vi "RFSA List Mode Frequency Sweep.vi"() -> ()   [LabVIEW 2017]
doc: "Demonstrates the basics of RF list mode using the RF vector signal analyzer. The example shows how to configure the device for RF list mode and how to create a configuration list and configuration list steps. It uses RF list mode to vary the I/Q carrier frequency and reference level across different steps that advance on a hardware timer edge."
uses:
  <instrlib>/niRFSA/niRFSA.llb/niRFSA Acquisition Types.ctl
  <instrlib>/niRFSA/niRFSA.llb/niRFSA Trigger Terminals.ctl
  <vilib>/Utility/error.llb/DialogType.ctl
  <vilib>/Analysis/1siggen.llb/Ramp Pattern by Samples.vi
  <instrlib>/niRFSA/niRFSA.llb/niRFSA Configure Digital Edge Advance Trigger.vi
  <instrlib>/niRFSA/niRFSA.llb/niRFSA Fetch IQ (1D Complex Cluster NRec 1Chan).vi
  <instrlib>/niRFSA/niRFSA.llb/niRFSA Get IQ Components (Complex Cluster).vi
  <vilib>/Analysis/NI_AALBase.lvlib
panel:
  in  "Frequency Settling (s)":dbl=0.006 format="%#_6p"
  in  "Reference Level (dBm)":dbl caption="Reference Level Ramp Start (dBm)" format="%.2g"
  out "Q Data":cluster{"t0":dbl, "dt":dbl, "Y":dbl[]}[](graph)
  out "I Data":cluster{"t0":dbl, "dt":dbl, "Y":dbl[]}[](graph)
  in  "Timer Event Interval (s)":dbl=0.001 format="%#_6p"
  in  "Carrier Frequency Ramp Start (Hz)":dbl=990000000.0 format="%#.3p"
  in  "Carrier Frequency Ramp End (Hz)":dbl=1010000000.0 format="%#.3p"
  in  "Number of Steps/Records":dbl=10.0
  in  "Samples per Step/Record":dbl=10000.0 format="%#_6p"
  in  "IQ Rate (S/s)":dbl=10000000.0 format="%#_6p"
  in  "Resource Name":refnum<k15>="RFSA"
  # "Overview: Demonstrates the basics of RF list mode using the RF vector signal analyzer. \nRequirements: NI-RFSA\nInstructions:\n1. Change the Resource Name to your device.\n2. Run the VI."
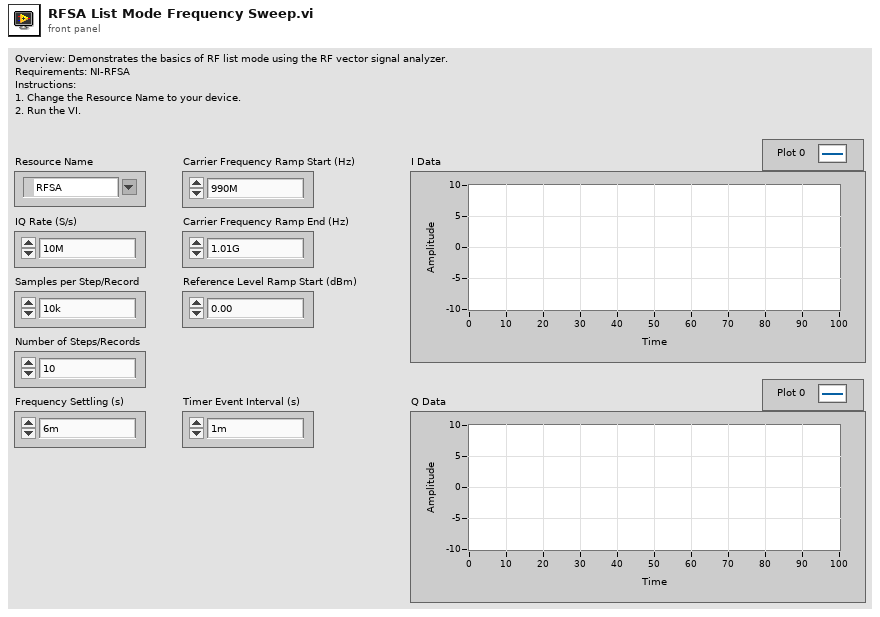
[diagram p1: front panel]
types:
  T1 = typedef "DialogType.ctl" = u16
  T2 = typedef "niRFSA Trigger Terminals.ctl" = string
  T3 = typedef "niRFSA Acquisition Types.ctl" = i32
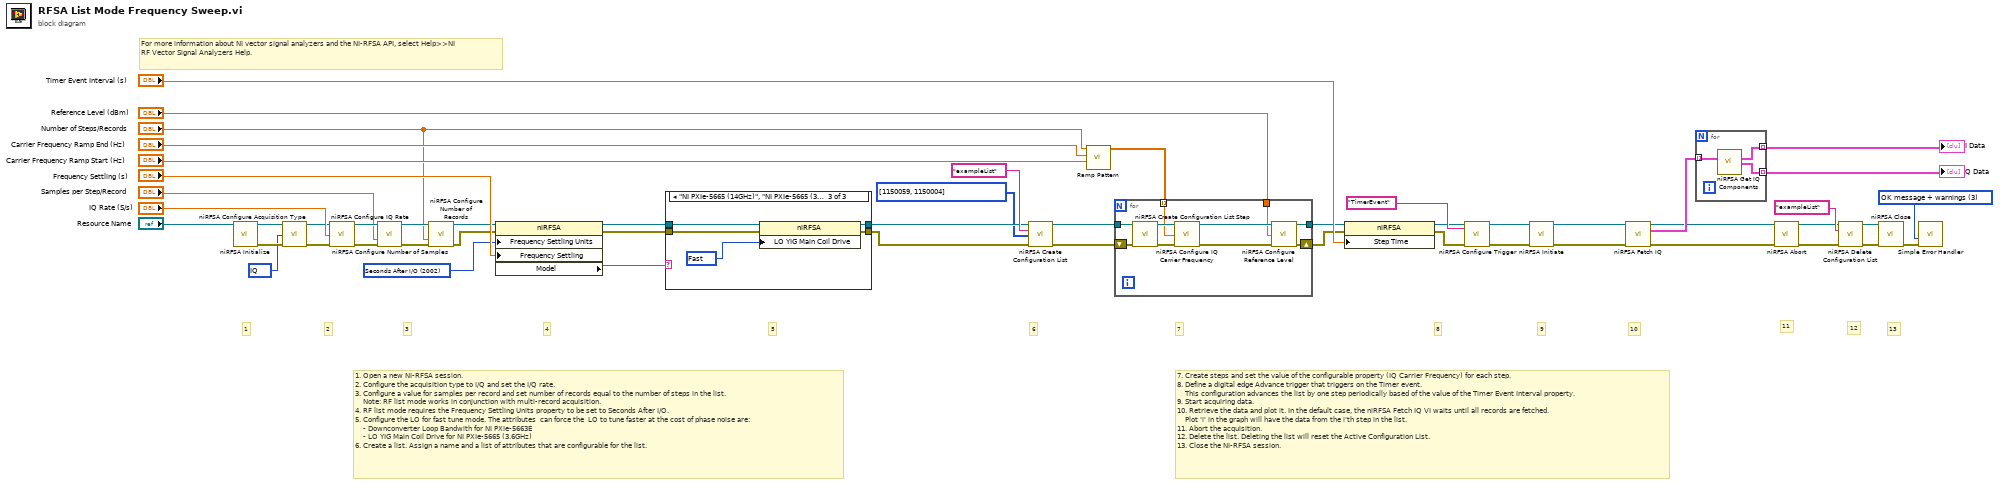
[diagram p0: block diagram]
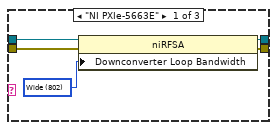
[diagram p2: hidden frame]
diagram:
  w5 = i32[] [1150059, 1150004] items=["Channel Coupling"=1150149, "DDC Reference Trigger Override"=1150164, "Device Instantaneous Bandwidth"=1150125, "Downconverter Center Frequency"=1150082, "Downconverter Frequency Offset"=1150203, "Downconverter Preselector Enabled"=1150132, "External Gain"=1150094, "Frequency Settling"=1150088, "IF Filter Bandwidth"=1150205, "IF Output Power Level"=1150130, "IF Output Power Level Offset"=1150131, "IQ Carrier Frequency"=1150059, "IQ In Port Carrier Frequency"=1150181, "IQ In Port Vertical Range"=1150183, "IQ Power Edge Level"=1150056, "Low Frequency Bypass Enabled"=1150207, "Mechanical Attenuation"=1150128, "Mechanical Attenuator Enabled"=1150081, "Minimum ACPR"=1150142, "Minimum Reconfiguration Time"=1150165, "Number of Samples"=1150009, "OSP Data Scaling Factor"=1150151, "Reference Level"=1150004, "RF Attenuation"=1150005, "RF Preamp Enabled"=1150129, "Timer Event Interval"=1150096] ("Configuration List Properties")
  w19 = T1 3 items=["no dialog", "OK message", "continue or stop message", "OK message + warnings", "continue/stop + warnings"] ("type of dialog (OK msg:1)")
  w1 = 2002 items=["PPM"=2000, "Seconds After Lock"=2001, "Seconds After I/O"=2002] ("Advanced:NI 5601:Frequency Settling Units")
  w49 = T3 100 items=["IQ"=100, "Spectrum"=101] ("acquisition type")
  # "For more information about NI vector signal analyzers and the NI-RFSA API, select Help>>NI  RF Vector Signal Analyzers Help."
  # "11"
  # "12"
  # "4"
  # "3"
  # "7. Create steps and set the value of the configurable property (IQ Carrier Frequency) for each step.\n8. Define a digital edge Advance trigger that triggers on the Timer event.\n    This configuration advances the list by one step periodically based of the value of the Timer Event Interval property.\n9. Start acquiring data.\n10. Retrieve the data and plot it. In the default case, the niRFSA Fetch IQ VI waits until all records are fetched. \n    Plot 'i' in the graph will have the data from the i'th step in the list.\n11. Abort the acquisition.\n12. Delete the list. Deleting the list will reset the Active Configuration List.\n13. Close the NI-RFSA session."
  # "1"
  # "13"
  # "10"
  # "8"
  # "1. Open a new NI-RFSA session.\n2. Configure the acquisition type to I/Q and set the I/Q rate.\n3. Configure a value for samples per record and set number of records equal to the number of steps in the list.\n    Note: RF list mode works in conjunction with multi-record acquisition.\n4. RF list mode requires the Frequency Settling Units property to be set to Seconds After I/O.\n5. Configure the LO for fast tune mode. The attributes  can force the  LO to tune faster at the cost of phase noise are: \n    - Downconverter Loop Bandwith for NI PXIe-5663E\n    - LO YIG Main Coil Drive for NI PXIe-5665 (3.6GHz)\n6. Create a list. Assign a name and a list of attributes that are configurable for the list."
  # "9"
  # "7"
  # "6"
  # "5"
  # "2"
  n1 = call <instrlib>:"niRFSA Initialize.vi"("resource name"="Resource Name") -> ("instrument handle out"=w51:refnum<k15>, "error out"=w50:errorcluster)  [unwired: 13 in]
  n2 = call <instrlib>:"niRFSA Configure Acquisition Type.vi"("instrument handle"=w51, "acquisition type"=w49, "error in"=w50) -> ("instrument handle out"=w28:refnum<k15>, "error out"=w27:errorcluster)  [unwired: 11 in]
  n3 = call <instrlib>:"niRFSA Configure IQ Rate.vi"("instrument handle"=w28, "IQ rate (S/s)"="IQ Rate (S/s)", "error in"=w27) -> ("instrument handle out"=w47:refnum<k15>, "error out"=w46:errorcluster)  [unwired: 11 in]
  n4 = call <instrlib>:"niRFSA Configure Number of Samples.vi"("instrument handle"=w47, "samples per record"="Samples per Step/Record", "error in"=w46) -> ("instrument handle out"=w44:refnum<k15>, "error out"=w43:errorcluster)  [unwired: 11 in]
  n5 = call <instrlib>:"niRFSA Configure Number of Records.vi"("instrument handle"=w44, "number of records"="Number of Steps/Records", "error in"=w43) -> ("instrument handle out"=w17:refnum<k15>, "error out"=w16:errorcluster)  [unwired: 11 in]
  n6 = property class="niRFSA"(reference=w17, error in=w16, "Frequency Settling Units"=w1, "Frequency Settling"="Frequency Settling (s)") -> (reference out=w15:refnum<k15>, error out=w14:errorcluster, "Model"=w11:string)
  n7 = case shown="\"NI PXIe-5665 (14GHz)\", \"NI PXIe-5665 (3.6GHz)\", \"NI PXIe-5667 (3.6GHz)\", \"NI PXIe-5667 (7GHz)\"" w11 {
    tunnel: w15 -> [w57 w59 w64]
    tunnel: w14 -> [w56 w58 w63]
    tunnel: [w55 w59 w62] -> w13
    tunnel: [w54 w58 w61] -> w12
    frame "NI PXIe-5663E" {
      w53 = 802 items=["Narrow"=800, "Medium"=801, "Wide"=802] ("Signal Path:NI 5600:Downconverter Loop Bandwidth")
      n8 = property class="niRFSA"(reference=w57, error in=w56, "Downconverter Loop Bandwidth"=w53) -> (reference out=w55:refnum<k15>, error out=w54:errorcluster)
    }
    frame Default {
    }
    frame "NI PXIe-5665 (14GHz)", "NI PXIe-5665 (3.6GHz)", "NI PXIe-5667 (3.6GHz)", "NI PXIe-5667 (7GHz)" {
      w60 = 2401 items=["Normal"=2400, "Fast"=2401] ("Signal Path:NI 5603:LO YIG Main Coil Drive")
      n9 = property class="niRFSA"(reference=w64, error in=w63, "LO YIG Main Coil Drive"=w60) -> (reference out=w62:refnum<k15>, error out=w61:errorcluster)
    }
  }
  n10 = call <instrlib>:"niRFSA Create Configuration List.vi"("instrument handle"=w13, "list name"="exampleList", "Configuration List Properties"=w5, "error in"=w12) -> ("instrument handle out"=w41:refnum<k15>, "error out"=w40:errorcluster)  [unwired: 10 in]
  n11 = call-poly <vilib>:"Ramp Pattern.vi"("start"="Carrier Frequency Ramp Start (Hz)", "end"="Carrier Frequency Ramp End (Hz)", "samples"="Number of Steps/Records") -> ("Ramp Pattern"=w39:dbl[])  [unwired: 7 in, 1 out]
  n12 = for {
    tunnel: w41 -> [w74]
    tunnel: w39 -> [w71] mode=indexing
    tunnel: [w67] -> w26
    shift-right: [w66] -> w25
    shift-left: w40 -> [w73]
    tunnel: "Reference Level (dBm)" -> [w65]
    n13 = call <instrlib>:"niRFSA Create Configuration List Step.vi"("instrument handle"=w74, "error in"=w73) -> ("instrument handle out"=w72:refnum<k15>, "error out"=w70:errorcluster)  [unwired: 12 in]
    n14 = call <instrlib>:"niRFSA Configure IQ Carrier Frequency.vi"("instrument handle"=w72, "carrier frequency"=w71, "error in"=w70) -> ("instrument handle out"=w69:refnum<k15>, "error out"=w68:errorcluster)  [unwired: 11 in]
    n15 = call <instrlib>:"niRFSA Configure Reference Level.vi"("instrument handle"=w69, "reference level (dBm)"=w65, "error in"=w68) -> ("instrument handle out"=w67:refnum<k15>, "error out"=w66:errorcluster)  [unwired: 11 in]
  }
  n16 = property class="niRFSA"(reference=w26, error in=w25, "Step Time"="Timer Event Interval (s)") -> (reference out=w23:refnum<k15>, error out=w22:errorcluster)
  n17 = call-poly <instrlib>:"niRFSA Configure Trigger.vi"("instrument handle"=w23, "source"=T2 "TimerEvent", "error in"=w22) -> ("instrument handle out"=w21:refnum<k15>, "error out"=w20:errorcluster)  [unwired: 11 in]
  n18 = call <instrlib>:"niRFSA Initiate.vi"("instrument handle"=w21, "error in"=w20) -> ("instrument handle out"=w34:refnum<k15>, "error out"=w33:errorcluster)  [unwired: 12 in]
  n19 = call-poly <instrlib>:"niRFSA Fetch IQ.vi"("instrument handle"=w34, "error in"=w33) -> ("instrument handle out"=w9:refnum<k15>, "data"=w30:cluster{"t0":dbl, "dt":dbl, "Y":cdb[]}[], "error out"=w8:errorcluster)  [unwired: 11 in]
  n20 = for {
    tunnel: [w77] -> w32 mode=indexing
    tunnel: [w76] -> w31 mode=indexing
    tunnel: w30 -> [w75] mode=indexing
    n21 = call-poly <instrlib>:"niRFSA Get IQ Components.vi"("data"=w75) -> ("I"=w77:cluster{"t0":dbl, "dt":dbl, "Y":dbl[]}, "Q"=w76:cluster{"t0":dbl, "dt":dbl, "Y":dbl[]})  [unwired: 11 in, 2 out]
  }
  "I Data" <- w32
  "Q Data" <- w31
  n22 = call <instrlib>:"niRFSA Abort.vi"("instrument handle"=w9, "error in"=w8) -> ("instrument handle out"=w6:refnum<k15>, "error out"=w7:errorcluster)  [unwired: 12 in]
  n23 = call <instrlib>:"niRFSA Delete Configuration List.vi"("instrument handle"=w6, "list name"="exampleList", "error in"=w7) -> ("instrument handle out"=w3:refnum<k15>, "error out"=w4:errorcluster)  [unwired: 11 in]
  n24 = call <instrlib>:"niRFSA Close.vi"("instrument handle"=w3, "error in"=w4) -> ("error out"=w18:errorcluster)  [unwired: 13 in]
  n25 = call <vilib>:"Simple Error Handler.vi"("type of dialog (OK msg:1)"=w19, "error in (no error)"=w18) -> ()  [unwired: 3 in, 5 out]
